vi "Add Control in Result.vi"(0 "result cluster":refnum<vi>, 1 "output clusters in":string[](array[string]), 5 "vi reference":refnum<vi>, 7 "ctl refnum":refnum<vi>, 11 "error in":errorcluster) -> (4 "output clusters out":string[](array[string]), 15 "error out":errorcluster)   [LabVIEW 2021, in "Converter.lvlib"]
uses:
  Converter.lvlib
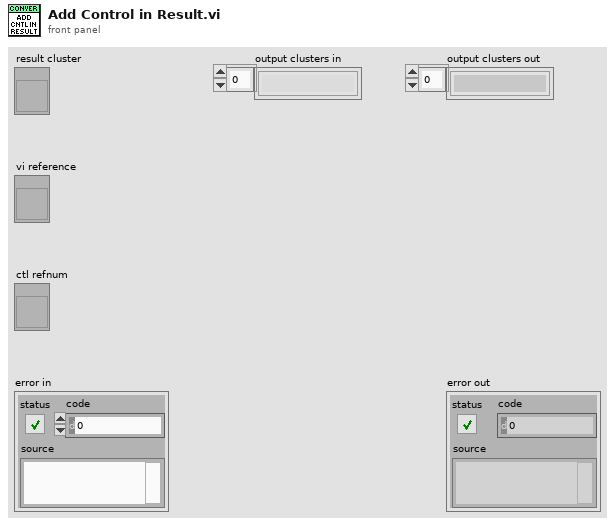
[diagram p1: front panel]
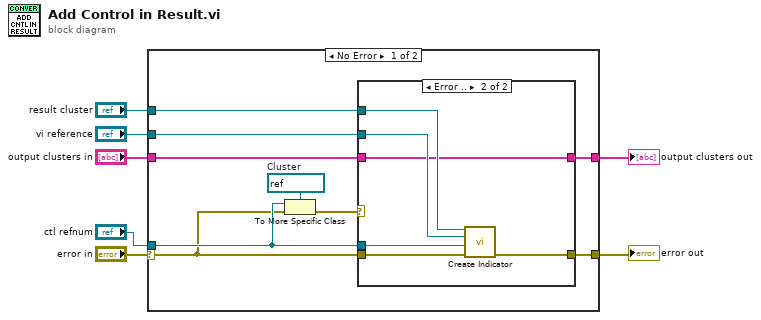
[diagram p0: block diagram]
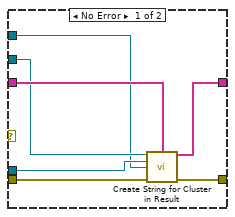
[diagram p2: hidden frame]
diagram:
  n1 = case shown="No Error" "error in" {
    selector: "error in" -> [w8 w30]
    tunnel: "output clusters in" -> [w16 _]
    tunnel: [w15 _] -> w6
    tunnel: "ctl refnum" -> [w14 _]
    tunnel: "vi reference" -> [w11 _]
    tunnel: [w10 w30] -> w3
    tunnel: "result cluster" -> [w9 _]
    frame No Error {
      w12 = refnum<vi> refnum  # Cluster
      n2 = To More Specific Class(target class=w12, reference=w14, error in=w8) -> (error out=w13:errorcluster)  [unwired: 1 out]
      n3 = case shown="Error .." w13 {
        tunnel: w9 -> [w18 w29]
        tunnel: [w17 w28] -> w10
        tunnel: w11 -> [w20 w27]
        tunnel: w14 -> [w19 w26]
        tunnel: w8 -> [w23 w25]
        tunnel: [w22 w24] -> w15
        tunnel: w16 -> [w21 w24]
        frame No Error {
          n4 = call "Create String for Cluster in Result.vi"("vi reference"=w20, "output cluster[]"=w21, "ctl refnum"=w19, "result cluster"=w18, "error in"=w23) -> ("output clusters"=w22:string[], "error out"=w17:errorcluster)  [unwired: 9 in]
        }
        frame Error {
          n5 = call "Create Indicator.vi"("result cluster"=w29, "vi reference"=w27, "ctl refnum"=w26, "error in"=w25) -> ("error out"=w28:errorcluster)  [unwired: 11 in]
        }
      }
    }
    frame Error {
    }
  }
  "output clusters out" <- w6
  "error out" <- w3
